vi "Variant to KVP.vi"(10 "Variant":variant) -> (2 "KVP Dictionary":variant)   [LabVIEW 2013, in "OpenVariant.lvlib"]
doc: "This VI takes a default value as the input and replaces it recursively (cluster, array) with values found in key value pair arrays."
uses:
  OpenVariant.lvlib
  Conversions/OpenConvert.lvlib
  TypeDescriptor/OpenDescriptor.lvlib
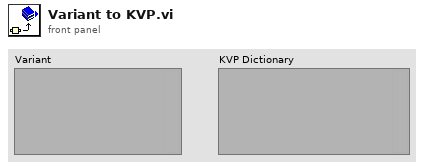
[diagram p1: front panel]
types:
  T1 = typedef "OpenDescriptor.lvlib/OpenDescriptor -- cluster.ctl" = cluster{"type descriptor":i16[], "name":string, "class":string, "data string":string}
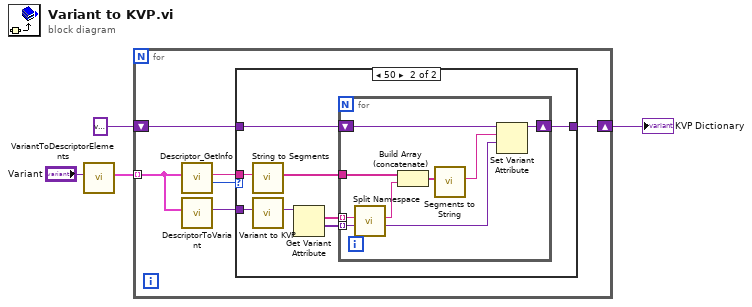
[diagram p0: block diagram]
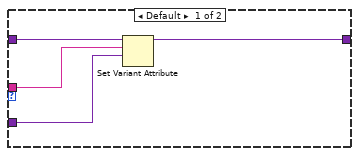
[diagram p2: hidden frame]
diagram:
  n1 = call "VariantToDescriptorElements.vi"("Variant"="Variant") -> ("Descriptors"=w1:T1[])  [unwired: 9 in, 1 out]
  n2 = for {
    shift-right: [w9] -> w4
    shift-left: variant ("Variant") -> [w10]
    tunnel: w1 -> [w6] mode=indexing
    n3 = call "Descriptor_GetInfo.vi"("Descriptor"=w6) -> ("Type"=w8:u8, "name"=w7:string)  [unwired: 8 in]
    n4 = call "DescriptorToVariant.vi"("Descriptor"=w6) -> ("Variant"=w5:variant)  [unwired: 10 in]
    n5 = case shown="50" w8 {
      tunnel: w7 -> [w13 w17]
      tunnel: w10 -> [w14 w22]
      tunnel: [w12 w21] -> w9
      tunnel: w5 -> [w11 w15]
      frame Default {
        n6 = Set Variant Attribute(Variant=w14, name=w13, value=w11) -> (Variant out=w12:variant)  [unwired: 1 in, 2 out]
      }
      frame 80 {
        n7 = call "String to Segments.vi"("String"=w17) -> ("Segments"=w16:string[])  [unwired: 9 in, 1 out]
        n8 = call "Variant to KVP.vi"("Variant"=w15) -> ("KVP Dictionary"=w20:variant)  [unwired: 10 in]
        n9 = Get Variant Attribute(Variant=w20) -> (names=w19:string[], values=w18:variant[])  [unwired: 3 in, 2 out]
        n10 = for {
          shift-right: [w30] -> w21
          shift-left: w22 -> [w29]
          tunnel: w19 -> [w25] mode=indexing
          tunnel: w18 -> [w28] mode=indexing
          tunnel: w16 -> [w23]
          n11 = call "Split Namespace.vi"("Namespaced String"=w25) -> ("String"=w24:string)  [unwired: 9 in, 1 out]
          n12 = Build Array (concatenate)(w23, w24) -> (w27:string[])
          n13 = call "Segments to String.vi"("Segments"=w27) -> ("String"=w26:string)  [unwired: 10 in]
          n14 = Set Variant Attribute(Variant=w29, name=w26, value=w28) -> (Variant out=w30:variant)  [unwired: 1 in, 2 out]
        }
      }
    }
  }
  "KVP Dictionary" <- w4
